vi "AlliGator Load Piccolo hist .bin FLI Dataset Prelude.vi"(8 "error in (no error)":errorcluster, 11 "File Path in":path) -> (0 "error out":errorcluster, 1 "Metdata":string, 2 "FLI Data File Information":T1, 3 "File Path out":path, 4 "Data Description":string)   [LabVIEW 2021, in "AlliGator Files.lvlib"]
doc: "Preliminary loading steps for Piccolo .bin files."
uses:
  AlliGator Files.lvlib
  HDF5/AlliGator FLI Data File Information.ctl
  Phasor/Phasor Fluorescence Lifetime Parameters v3.ctl
  AlliGator FLI Dataset Type.ctl
  AlliGator Piccolo hist .bin Dataset Information.ctl
  AlliGator Piccolo hist BIN File Information.ctl
  AlliGator Load Single Gate Image from Piccolo hist .bin File.vi
  Phasor/Phasor.lvlib
  HDF5/AlliGator HDF5.lvlib
panel:
  # "see the AlliGator License on the block diagram (Ctrl+E or Window:Show Block Diagram)"
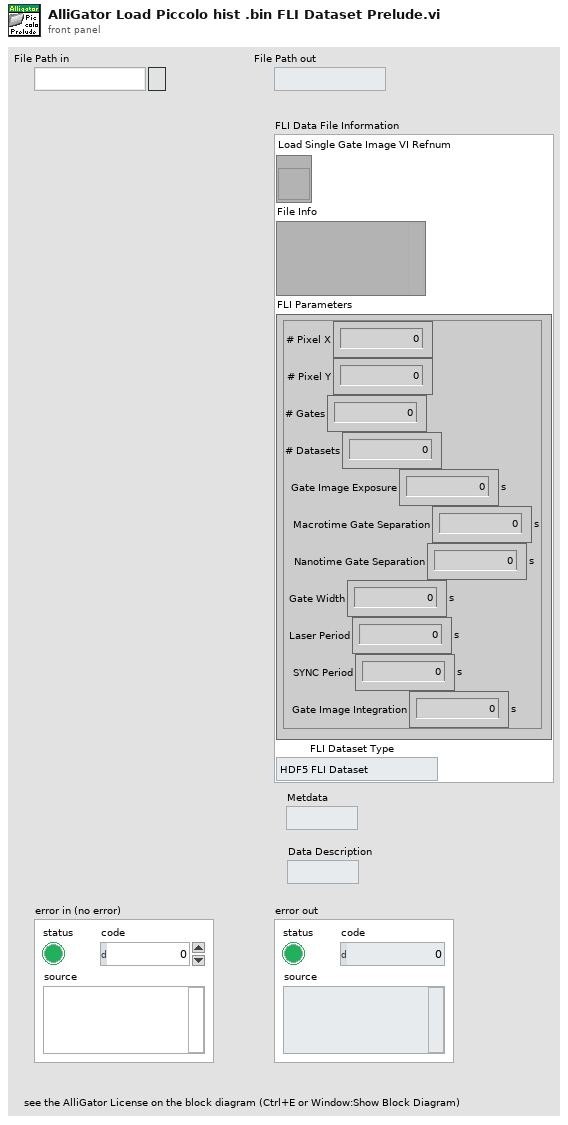
[diagram p1: front panel]
types:
  T1 = typedef "AlliGator HDF5.lvlib/AlliGator FLI Data File Information.ctl" = cluster{"Load Single Gate Image VI Refnum":refnum<vi>, "File Info":variant, "FLI Parameters":T2, "FLI Dataset Type":T3}
  T2 = typedef "Phasor.lvlib/Phasor Fluorescence Lifetime Parameters v3.ctl" = cluster{"# Pixel X":i32, "# Pixel Y":i32, "# Gates":i32, "# Datasets":i32, "Gate Image Exposure":dbl[unit], "Macrotime Gate Separation":dbl[unit], "Nanotime Gate Separation":dbl[unit], "Gate Width":dbl[unit], "Laser Period":dbl[unit], "SYNC Period":dbl[unit], "Gate Image Integration":dbl[unit]}
  T3 = typedef "AlliGator Files.lvlib/AlliGator FLI Dataset Type.ctl" = enum16{"HDF5 FLI Dataset", "Gate Image Folder", ".sdt FLI Dataset (Becker & Hickl)", ".ptu FLI Dataset (PicoQuant)", "SS1 FLI Dataset", "SS2 FLI Dataset", "I/m/phi Dataset", ".bin FLI Dataset (PicoQuant Binned)", ".bin FLI Dataset (Piccolo Binned)"}
  T4 = typedef "AlliGator Files.lvlib/AlliGator Piccolo hist .bin Dataset Information.ctl" = cluster{"File Path":path, "Piccolo hist BIN dataset Information":T5}
  T5 = typedef "AlliGator Files.lvlib/AlliGator Piccolo hist BIN File Information.ctl" = cluster{"# Pixels X":i32, "# Pixels Y":i32, "# TCSPC Bins":i32, "Temporal Resolution":dbl[unit]}
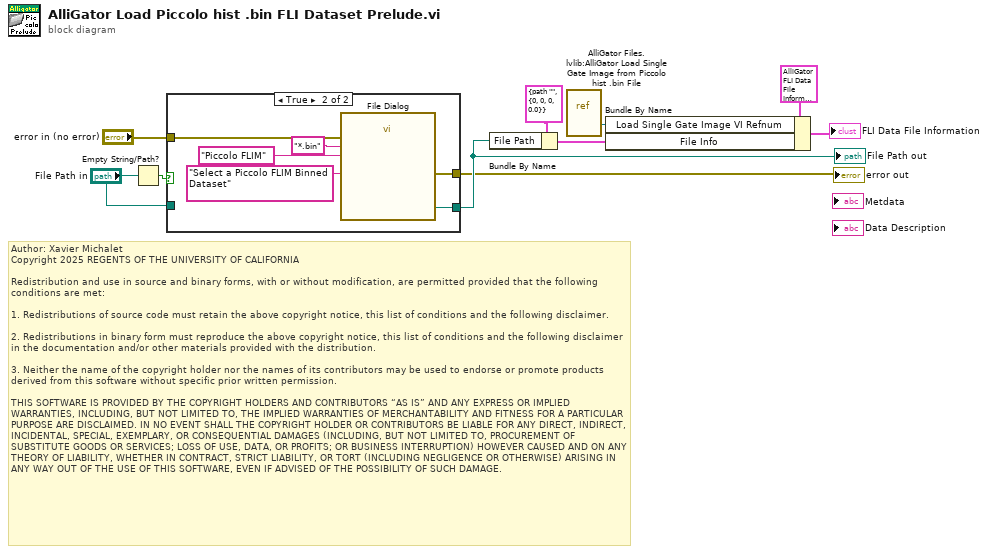
[diagram p0: block diagram]
diagram:
  # "Author: Xavier Michalet\nCopyright 2025 REGENTS OF THE UNIVERSITY OF CALIFORNIA\n\nRedistribution and use in source and binary forms, with or without modification, are permitted provided that the following conditions are met:\n\n1. Redistributions of source code must retain the above copyright notice, this list of conditions and the following disclaimer.\n\n2. Redistributions in binary form must reproduce the above copyright notice, this list of conditions and the following disclaimer in the documentation and/or other materials provided with the distribution.\n\n3. Neither the name of the copyright holder nor the names of its contributors may be used to endorse or promote products derived from this software without specific prior written permission.\n\nTHIS SOFTWARE IS PROVIDED BY THE COPYRIGHT HOLDERS AND CONTRIBUTORS “AS IS” AND ANY EXPRESS OR IMPLIED WARRANTIES, INCLUDING, BUT NOT LIMITED TO, THE IMPLIED WARRANTIES OF MERCHANTABILITY AND FITNESS FOR A PARTICULAR PURPOSE ARE DISCLAIMED. IN NO EVENT SHALL THE COPYRIGHT HOLDER OR CONTRIBUTORS BE LIABLE FOR ANY DIRECT, INDIRECT, INCIDENTAL, SPECIAL, EXEMPLARY, OR CONSEQUENTIAL DAMAGES (INCLUDING, BUT NOT LIMITED TO, PROCUREMENT OF SUBSTITUTE GOODS OR SERVICES; LOSS OF USE, DATA, OR PROFITS; OR BUSINESS INTERRUPTION) HOWEVER CAUSED AND ON ANY THEORY OF LIABILITY, WHETHER IN CONTRACT, STRICT LIABILITY, OR TORT (INCLUDING NEGLIGENCE OR OTHERWISE) ARISING IN ANY WAY OUT OF THE USE OF THIS SOFTWARE, EVEN IF ADVISED OF THE POSSIBILITY OF SUCH DAMAGE."
  n1 = Empty String/Path?(string/path="File Path in") -> (empty?=w10:bool)
  n2 = case shown="True" w10 {
    tunnel: "error in (no error)" -> [w11 w18]
    tunnel: [w12 w14] -> w4
    tunnel: [w11 w13] -> w1
    tunnel: "File Path in" -> [w12 _]
    frame False {
    }
    frame True {
      n3 = call "File Dialog"("prompt"="Select a Piccolo FLIM Binned Dataset", "error in"=w18, "pattern (all files)"="*.bin", "pattern label"="Piccolo FLIM") -> ("selected path"=w14:path, "error out"=w13:errorcluster)  [unwired: 8 in, 2 out]
    }
  }
  "error out" <- w1
  "File Path out" <- w4
  n4 = Bundle By Name(cluster=T4 {"File Path"=path "", "Piccolo hist BIN dataset Information"={"# Pixels X"=0, "# Pixels Y"=0, "# TCSPC Bins"=0, "Temporal Resolution"=0.0}} ("output cluster"), "File Path"=w4) -> (w3:T4)
  n5 = vi-ref "AlliGator Files.lvlib:AlliGator Load Single Gate Image from Piccolo hist .bin File.vi"() -> (w6:refnum<vi>)
  n6 = Bundle By Name(cluster=T1 {"Load Single Gate Image VI Refnum"=refnum, "File Info"=variant, "FLI Parameters"={"# Pixel X"=0, "# Pixel Y"=0, "# Gates"=0, "# Datasets"=0, "Gate Image Exposure"=0.0, "Macrotime Gate Separation"=0.0, "Nanotime Gate Separation"=0.0, "Gate Width"=0.0, "Laser Period"=0.0, "SYNC Period"=0.0, "Gate Image Integration"=0.0}, "FLI Dataset Type"=enum."HDF5 FLI Dataset"} ("FLI Data File Information"), "Load Single Gate Image VI Refnum"=w6, "File Info"=w3) -> (→"FLI Data File Information":T1)
